vi "test 2d array round trip.vi"() -> ()   [LabVIEW 2020, in "jki_python_data_tools.lvlib"]
uses:
  jki_python_data_tools.lvlib
  LabVIEW Data to Python String/LabVIEW Data to Python String (Variant).vi
panel:
  out "Array":cluster{i32[][]}[][](array[cluster])
  out "data 2":i32[][](array[numeric])
  out "Iteration Time (ms)":dbl
  in  "Iteration":i32
  out "error out":errorcluster
  out "data":i32[][](array[numeric])
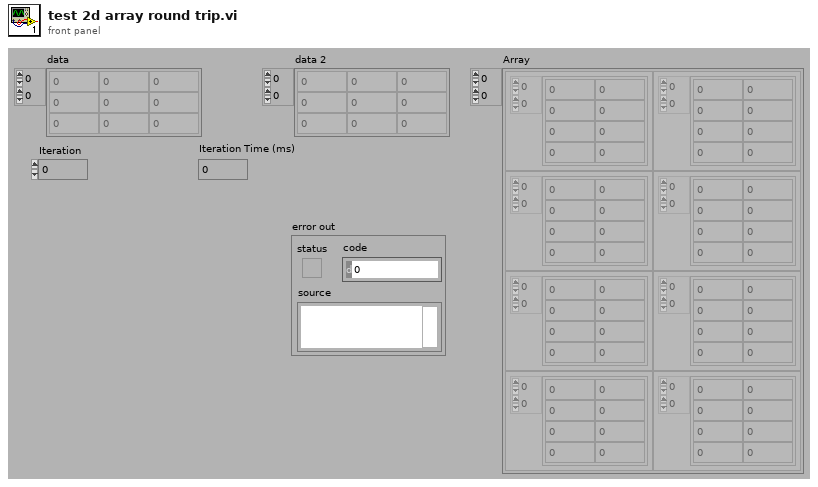
[diagram p1: front panel]
types:
  T1 = typedef "jki_python_data_tools.lvlib/Type Descriptor Enumeration__Py2LV.ctl" = enum8{"<Null>", "I8", "I16", "I32", "I64", "U8", "U16", "U32", "U64", "SGL", "DBL", "EXT", "CSG", "CDB", "CXT", "0x0F", "0x10", "0x11", "0x12", "0x13", "0x14", "Enum U8", "Enum U16", "Enum U32", "Enum U64", "SGL PQ", "DBL PQ", "EXT PQ", "CSG PQ", "CDB PQ", "CXT PQ", "0x1F", "0x20", "Boolean", "0x22", "0x23", "0x24", "0x25", "0x26", "0x27", "0x28", "0x29", "0x2A", "0x2B", "0x2C", "0x2D", "0x2E", "0x2F", "String", "0x31", "Path", "Pict", "0x34", "0x35", "0x36", "DAQ", "0x38", "0x39", "0x3A", "0x3B", "0x3C", "0x3D", "0x3E", "0x3F", "Array", "0x41", "0x42", "0x43", "0x44", "0x45", "0x46", "0x47", "0x48", "0x49", "0x4A", "0x4B", "0x4C", "0x4D", "0x4E", "0x4F", "Cluster", "0x51", "0x52", "Variant", "Waveform", "0x55", "0x56", "0x57", "0x58", "0x59", "0x5A", "0x5B", "0x5C", "0x5D", "0x5E", "0x5F", "0x60", "0x61", "0x62", "0x63", "0x64", "0x65", "0x66", "0x67", "0x68", "0x69", "0x6A", "0x6B", "0x6C", "0x6D", "0x6E", "0x6F", "Refnum"}
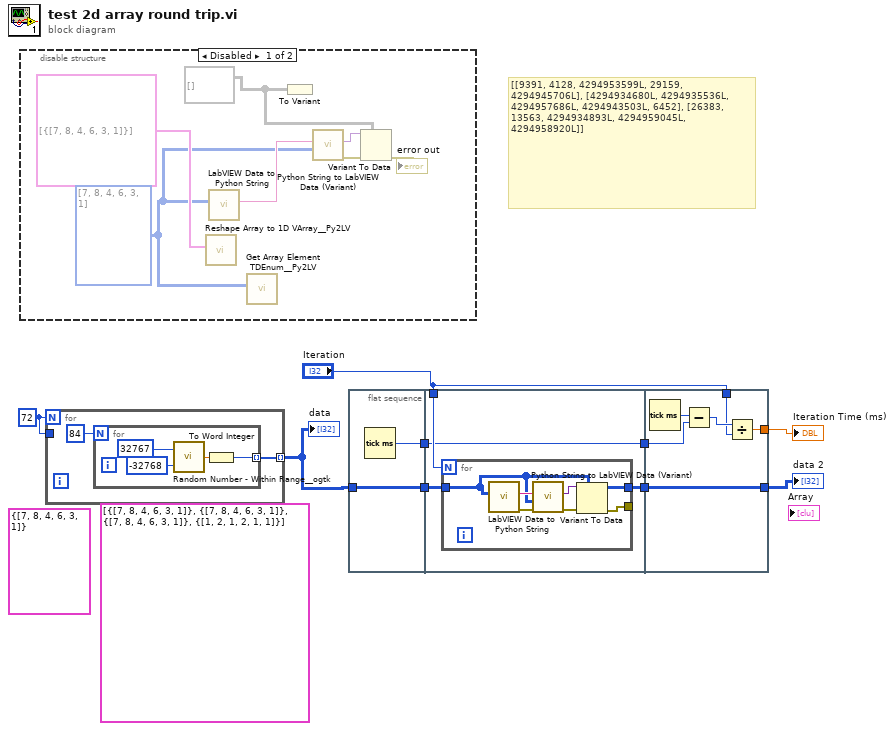
[diagram p0: block diagram]
diagram:
  (unwired) cluster{i32[][]} {[[7, 8], [4, 6], [3, 1]]}
  (unwired) cluster{i32[][]}[][] [[{[[7, 8], [4, 6], [3, 1]]}, {[[7, 8], [4, 6], [3, 1]]}], [{[[7, 8], [4, 6], [3, 1]]}, {[[1, 2], [1, 2], [1, 1]]}]]
  w9 = 72
  # "[[9391, 4128, 4294953599L, 29159, 4294945706L], [4294934680L, 4294935536L, 4294957686L, 4294943503L, 6452], [26383, 13563, 4294934893L, 4294959045L, 4294958920L]]"
  n1 = disable-structure shown="Disabled" {
    frame Disabled {
      w10 = void[][] [] ("data")
      w11 = i32[][] [[7, 8], [4, 6], [3, 1]]
      n2 = call "Reshape Array to 1D VArray__Py2LV.vi"("MultiD Array"=cluster{i32[][]}[] [{[[7, 8], [4, 6], [3, 1]]}]) -> ("1D VArray"=w18:variant)  [unwired: 8 in, 2 out]
      n3 = call-poly "LabVIEW Data to Python String.vi"("LabVIEW Data"=w11) -> ("Python String"=w15:string)  [unwired: 9 in, 1 out]
      n4 = call "Get Array Element TDEnum__Py2LV.vi"("Array"=w11) -> ("Element Type"=w17:T1)  [unwired: 9 in, 1 out]
      n5 = To Variant(anything=w10) -> ()  [unwired: 1 out]
      n6 = call "Python String to LabVIEW Data (Variant).vi"("type"=w11, "Python String"=w15) -> ("error out"=w14:errorcluster, "LabVIEW Data"=w13:variant)  [unwired: 8 in]
      n7 = Variant To Data(error in=w14, type=w10, Variant=w13) -> (error out=→"error out":errorcluster)  [unwired: 1 out]
    }
    frame Enabled {
    }
  }
  n8 = for {
    N: w9 -> [_]
    tunnel: w9 -> [_]
    tunnel: [w20] -> w2 mode=indexing
    n9 = for {
      N: 84 -> [_]
      tunnel: [w21] -> w20 mode=indexing
      n10 = call <userlib>:"Random Number - Within Range__ogtk.vi"("High (1.00)"=i16 32767, "Low (0.00)"=i16 -32768) -> ("Random Number"=w22:dbl)  [unwired: 3 in]
      n11 = To Word Integer(number=w22) -> (16bit integer=w21:i16)
    }
  }
  "data" <- w2
  n12 = flat-sequence {
    tunnel: w2 -> [w25]
    tunnel: [w26] -> w8
    tunnel: [w25] -> w3
    tunnel: [w30] -> w7
    tunnel: "Iteration" -> [w29]
    tunnel: w8 -> [w28]
    tunnel: [w28] -> w6
    tunnel: w3 -> [w27]
    tunnel: [w43] -> w1
    tunnel: w7 -> [w43]
    tunnel: w6 -> [w41]
    tunnel: "Iteration" -> [w39]
    tunnel: [w38] -> w5
    frame #0 {
      n13 = Tick Count (ms)() -> (millisecond timer value=w26:u32)
    }
    frame #1 {
      n14 = for {
        N: w29 -> [_]
        tunnel: [w31] -> w30
        tunnel: w27 -> [w32]
        tunnel: [w33] -> _
        n15 = call-poly "LabVIEW Data to Python String.vi"("LabVIEW Data"=w32) -> ("error out"=w37:errorcluster, "Python String"=w36:string)  [unwired: 9 in]
        n16 = call "Python String to LabVIEW Data (Variant).vi"("error in (no error)"=w37, "type"=w32, "Python String"=w36) -> ("error out"=w34:errorcluster, "LabVIEW Data"=w35:variant)  [unwired: 7 in]
        n17 = Variant To Data(error in=w34, type=w32, Variant=w35) -> (data=w31:i16[][], error out=w33:errorcluster)
      }
    }
    frame #2 {
      n18 = Tick Count (ms)() -> (millisecond timer value=w42:u32)
      n19 = Subtract(x=w42, y=w41) -> (x-y=w40:u32)
      n20 = Divide(x=w40, y=w39) -> (x/y=w38:dbl)
    }
  }
  "Iteration Time (ms)" <- w5
  "data 2" <- w1
